vi "Create Pattern Script(Data).vi"(8 "error in (no error)":errorcluster, 10 "Data":u8[](array[numeric]), 11 "BML Pattern Creater in":refnum<class "BML Pattern Creater.lvclass">) -> (0 "error out":errorcluster, 2 "String":string, 3 "BML Pattern Creater out":refnum<class "BML Pattern Creater.lvclass">)   [LabVIEW 2018, in "BML Pattern Creater.lvlib" / "BML Pattern Creater.lvclass"]
uses:
  BML Pattern Creater.lvclass
  Interfaces/Protocol Interface.lvlibp/Interfaces/Protocol Interface/Pin State.ctl
  Interfaces/Protocol Interface.lvlibp/Interfaces/Protocol Interface/Protocol Interface.lvclass
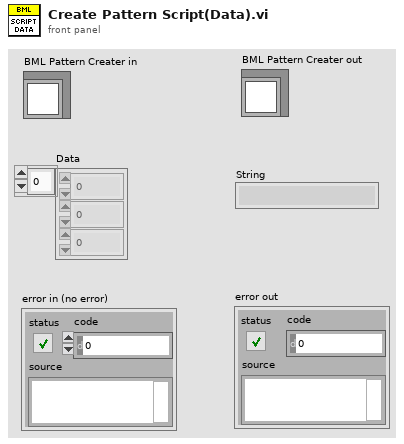
[diagram p1: front panel]
types:
  T1 = typedef "Protocol Interface.lvlibp/Protocol Interface.lvclass/Pin State.ctl" = enum16{"0", "1", "L", "H", "X", "V", "D", "M"}
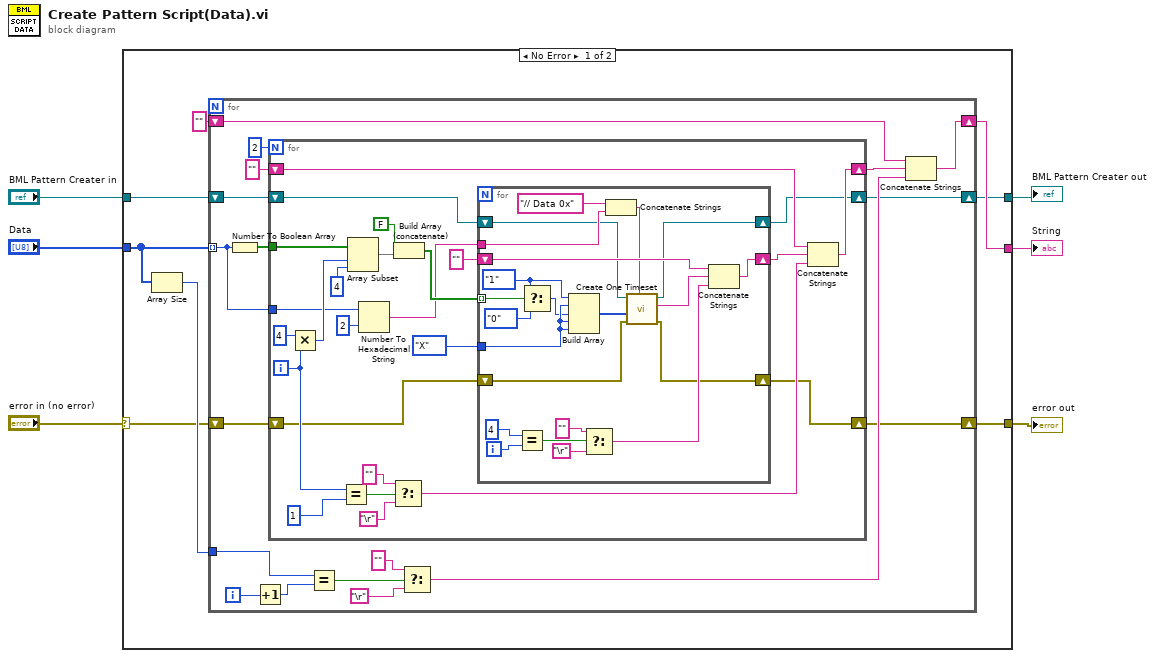
[diagram p0: block diagram]
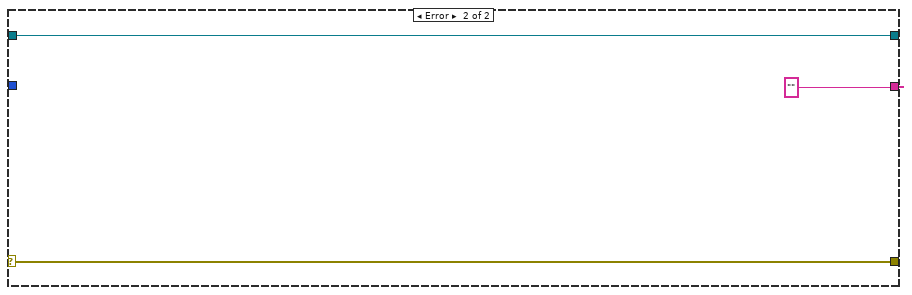
[diagram p2: hidden frame]
diagram:
  n1 = case shown="No Error" "error in (no error)" {
    selector: "error in (no error)" -> [w10 w81]
    tunnel: [w12 ""] -> w5
    tunnel: [w9 w81] -> w4
    tunnel: "Data" -> [w14 _]
    tunnel: "BML Pattern Creater in" -> [w8 w80]
    tunnel: [w7 w80] -> w1
    frame No Error {
      n2 = Array Size(array=w14) -> (size(s)=w13:i32)
      n3 = for {
        tunnel: w14 -> [w19] mode=indexing
        tunnel: w13 -> [w27]
        shift-right: [w21] -> w12
        shift-left: "" -> [w20]
        shift-right: [w17] -> w9
        shift-left: w10 -> [w18]
        shift-right: [w15] -> w7
        shift-left: w8 -> [w16]
        i -> [w29]
        n4 = Number To Boolean Array(number=w19) -> (Boolean array=w32:bool[])
        n5 = Increment(x=w29) -> (x+1=w28:i32)
        n6 = for {
          N: 2 -> [_]
          tunnel: w32 -> [w57]
          shift-right: [w43] -> w23
          shift-left: "" -> [w42]
          tunnel: w19 -> [w40]
          shift-right: [w35] -> w17
          shift-left: w18 -> [w36]
          shift-right: [w33] -> w15
          shift-left: w16 -> [w34]
          i -> [w50]
          n7 = Multiply(x=4 ("y"), y=w50) -> (x*y=w56:i32)
          n8 = Equal?(x=w50, y=1) -> (x = y?=w48:bool)
          n9 = Array Subset(array=w57, index=w56, length=4) -> (w55:bool[])
          n10 = Number To Hexadecimal String(1:i16 2 ("width (-)"), 2:w40) -> (0:w38:string)
          n11 = Select(t="", s=w48, f="\r") -> (s? t:f=w44:string)
          n12 = Build Array (concatenate)(FALSE, w55) -> (w52:bool[])
          n13 = for {
            tunnel: w52 -> [w79] mode=indexing
            shift-right: [w73] -> w45
            shift-left: "" -> [w72]
            tunnel: Pin_State."X" ("PinState") -> [w70]
            tunnel: w38 -> [w67]
            shift-right: [w60] -> w35
            shift-left: w36 -> [w61]
            shift-right: [w58] -> w33
            shift-left: w34 -> [w59]
            i -> [w78]
            w63 = Pin_State."1" ("PinState")
            n14 = Equal?(x=4, y=w78) -> (x = y?=w76:bool)
            n15 = Select(t=w63, s=w79, f=Pin_State."0" ("PinState")) -> (s? t:f=w69:T1)
            n16 = Build Array(w63, w70, w69, w70, w70) -> (w65:T1[])
            n17 = Select(t="", s=w76, f="\r") -> (s? t:f=w71:string)
            n18 = Concatenate Strings("// Data 0x" ("string"), w67) -> (w66:string)
            n19 = call-dynamic "Create One Timeset.vi"("Notes"=w66, "error in (no error)"=w61, "Pin State"=w65, "BML Pattern Creater in"=w59) -> ("error out"=w60:errorcluster, "string out"=w64:string, "BML Pattern Creater out"=w58:refnum<class "BML Pattern Creater.lvclass">)  [unwired: 5 in]
            n20 = Concatenate Strings(w72, w64, w71) -> (w73:string)
          }
          n21 = Concatenate Strings(w42, w45, w44) -> (w43:string)
        }
        n22 = Equal?(x=w27, y=w28) -> (x = y?=w24:bool)
        n23 = Select(t="", s=w24, f="\r") -> (s? t:f=w22:string)
        n24 = Concatenate Strings(w20, w23, w22) -> (w21:string)
      }
    }
    frame Error {
    }
  }
  "String" <- w5
  "error out" <- w4
  "BML Pattern Creater out" <- w1
